vi "make_plot_projection.vi"(0 "Plot Scene Object In":refnum<vi>, 2 "Surface Mesh In":refnum<vi>, 3 "Minimum":T1, 7 "Data Mesh Object In":refnum<vi>, 8 "Projection Properties":T3, 9 "Contour Object In":refnum<vi>, 11 "Normals Object In":refnum<vi>, 13 "PL Object In":refnum<vi>) -> (14 "Plot Scene Object Out":refnum<vi>, 16 "Surface Mesh Out":refnum<vi>)   [LabVIEW 2020, in "3DPC_SurfacePlot.xctl"]
uses:
  <vilib>/Native 3D Graph/xcontrol/3DPC_SurfacePlot.xctl
  <vilib>/Native 3D Graph/typedefs/prop_plot_projection.ctl
  <vilib>/Native 3D Graph/typedefs/range_cluster.ctl
  <vilib>/Native 3D Graph/typedefs/min_max.ctl
  <vilib>/picture/3D Picture Control/Object/Create Object (name).vi
  <vilib>/picture/3D Picture Control/NI_3D Picture Control.lvlib
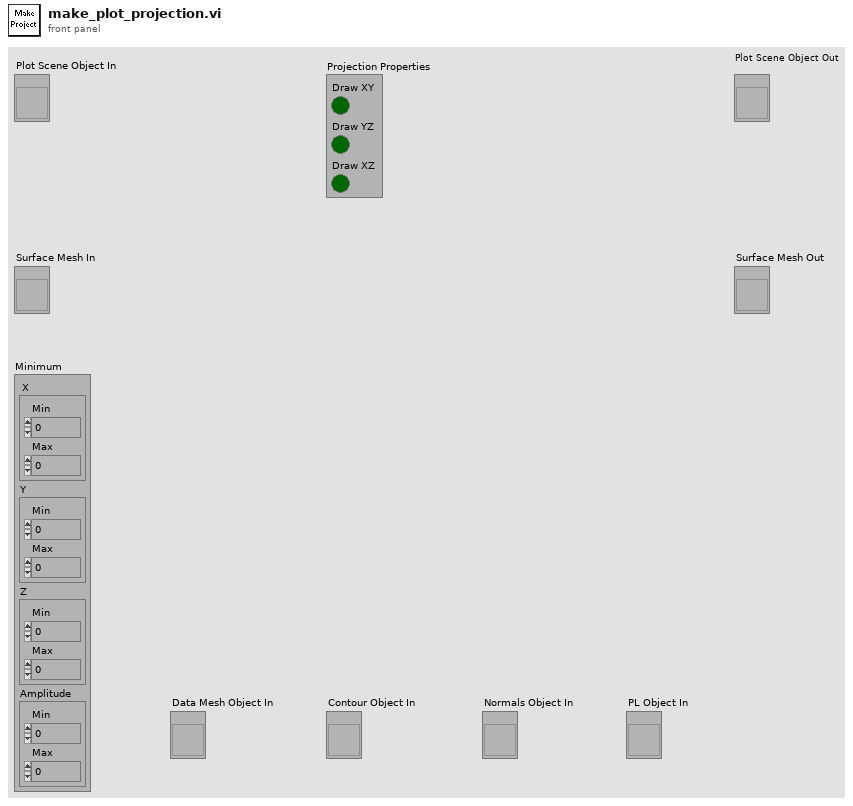
[diagram p1: front panel]
types:
  T1 = typedef "3DPC_SurfacePlot.xctl/range_cluster.ctl" = cluster{"X":T2, "Y":T2, "Z":T2, "Amplitude":T2}
  T2 = typedef "3DPC_SurfacePlot.xctl/min_max.ctl" = cluster{"Min":sgl, "Max":sgl}
  T3 = typedef "3DPC_SurfacePlot.xctl/prop_plot_projection.ctl" = cluster{"Draw XY":bool, "Draw YZ":bool, "Draw XZ":bool}
  T4 = enum16{"Inherit Value", "Points", "Wireframe", "Polygons"}
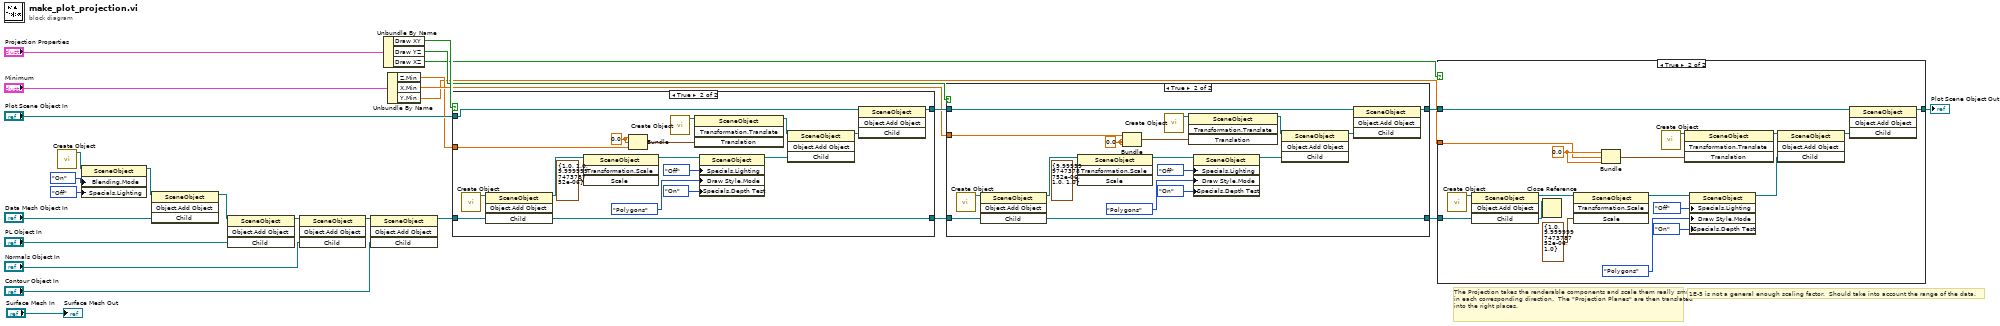
[diagram p0: block diagram]
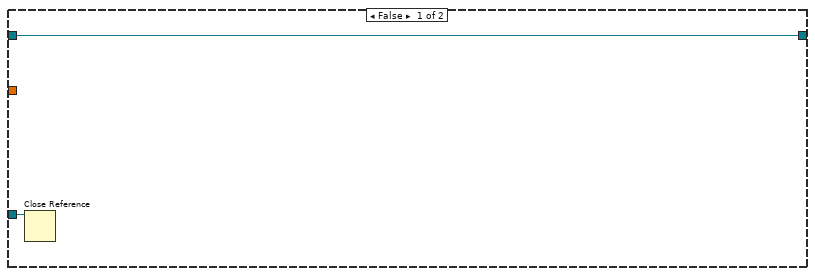
[diagram p2: hidden frame]
diagram:
  # "1E-5 is not a general enough scaling factor.  Should take into account the range of the data."
  # "The Projection takes the renderable components and scale them really small in each corresponding direction.  The \"Projection Planes\" are then translated into the right places."
  n1 = call-poly <vilib>:"Create Object.vi"() -> ("Scene:New Object"=w8:refnum<vi>)  [unwired: 10 in, 1 out]
  n2 = property class="SceneObject"(reference=w8, "Blending.Mode"=enum16{"Inherit Value", "Off", "On"}."On" ("Blending:Mode"), "Specials.Lighting"=enum16{"Inherit Value", "Off", "On"}."Off" ("Specials:Lighting")) -> (reference out=w9:refnum<vi>)  [unwired: 1 in, 1 out]
  n3 = invoke class="SceneObject" method="Object.Add Object"(reference=w9, "Child"="Data Mesh Object In") -> (reference out=w17:refnum<vi>)  [unwired: 2 in, 3 out]
  n4 = invoke class="SceneObject" method="Object.Add Object"(reference=w17, "Child"="PL Object In") -> (reference out=w16:refnum<vi>)  [unwired: 2 in, 3 out]
  n5 = invoke class="SceneObject" method="Object.Add Object"(reference=w16, "Child"="Normals Object In") -> (reference out=w15:refnum<vi>)  [unwired: 2 in, 3 out]
  n6 = invoke class="SceneObject" method="Object.Add Object"(reference=w15, "Child"="Contour Object In") -> (reference out=w10:refnum<vi>)  [unwired: 2 in, 3 out]
  n7 = Unbundle By Name("Projection Properties") -> ("Draw XY"=w21:bool, "Draw YZ"=w19:bool, "Draw XZ"=w18:bool)
  n8 = Unbundle By Name("Minimum") -> ("Z.Min"=w2:sgl, "X.Min"=w3:sgl, "Y.Min"=w1:sgl)
  n9 = case shown="True" w21 {
    tunnel: "Plot Scene Object In" -> [w29 w45]
    tunnel: [w29 w46] -> w24
    tunnel: [w28 w31] -> w25
    tunnel: w10 -> [w28 w32]
    tunnel: w2 -> [_ w30]
    frame False {
    }
    frame True {
      w36 = sgl 0.0 ("Minimum")
      n10 = call-poly <vilib>:"Create Object.vi"() -> ("Scene:New Object"=w47:refnum<vi>)  [unwired: 10 in, 1 out]
      n11 = invoke class="SceneObject" method="Object.Add Object"(reference=w47, "Child"=w32) -> (reference out=w41:refnum<vi>, "Child"=w31:refnum<vi>)  [unwired: 2 in, 2 out]
      n12 = invoke class="SceneObject" method="Transformation.Scale"(reference=w41, "Scale"=cluster{"X":sgl, "Y":sgl, "Z":sgl} {"X"=1.0, "Y"=1.0, "Z"=1e-05}) -> (reference out=w40:refnum<vi>)  [unwired: 2 in, 3 out]
      n13 = Bundle("Minimum"=w36, "Minimum"=w36, "Min"=w30) -> (w35:cluster{"Minimum":sgl, "Minimum":sgl, "Min":sgl})  [unwired: 1 out]
      n14 = call-poly <vilib>:"Create Object.vi"() -> ("Scene:New Object"=w38:refnum<vi>)  [unwired: 10 in, 1 out]
      n15 = invoke class="SceneObject" method="Transformation.Translate"(reference=w38, "Translation"=w35) -> (reference out=w37:refnum<vi>)  [unwired: 2 in, 3 out]
      n16 = property class="SceneObject"(reference=w40, "Specials.Lighting"=enum16{"Inherit Value", "Off", "On"}."Off" ("Specials:Lighting"), "Draw Style.Mode"=T4."Polygons" ("Draw Style:Mode"), "Specials.Depth Test"=enum16{"Inherit Value", "Off", "On"}."On" ("Specials:Depth Test")) -> (reference out=w34:refnum<vi>)  [unwired: 1 in, 1 out]
      n17 = invoke class="SceneObject" method="Object.Add Object"(reference=w37, "Child"=w34) -> (reference out=w33:refnum<vi>)  [unwired: 2 in, 3 out]
      n18 = invoke class="SceneObject" method="Object.Add Object"(reference=w45, "Child"=w33) -> (reference out=w46:refnum<vi>)  [unwired: 2 in, 3 out]
    }
  }
  n19 = case shown="True" w19 {
    tunnel: w24 -> [w49 w65]
    tunnel: [w49 w66] -> w22
    tunnel: w25 -> [w48 w61]
    tunnel: [w48 w55] -> w23
    tunnel: w3 -> [_ w50]
    frame False {
    }
    frame True {
      w51 = sgl 0.0 ("Minimum")
      n20 = call-poly <vilib>:"Create Object.vi"() -> ("Scene:New Object"=w67:refnum<vi>)  [unwired: 10 in, 1 out]
      n21 = invoke class="SceneObject" method="Object.Add Object"(reference=w67, "Child"=w61) -> (reference out=w60:refnum<vi>, "Child"=w55:refnum<vi>)  [unwired: 2 in, 2 out]
      n22 = invoke class="SceneObject" method="Transformation.Scale"(reference=w60, "Scale"=cluster{"X":sgl, "Y":sgl, "Z":sgl} {"X"=1e-05, "Y"=1.0, "Z"=1.0}) -> (reference out=w59:refnum<vi>)  [unwired: 2 in, 3 out]
      n23 = Bundle("Min"=w50, "Minimum"=w51, "Minimum"=w51) -> (w54:cluster{"Min":sgl, "Minimum":sgl, "Minimum":sgl})  [unwired: 1 out]
      n24 = call-poly <vilib>:"Create Object.vi"() -> ("Scene:New Object"=w53:refnum<vi>)  [unwired: 10 in, 1 out]
      n25 = invoke class="SceneObject" method="Transformation.Translate"(reference=w53, "Translation"=w54) -> (reference out=w52:refnum<vi>)  [unwired: 2 in, 3 out]
      n26 = property class="SceneObject"(reference=w59, "Specials.Lighting"=enum16{"Inherit Value", "Off", "On"}."Off" ("Specials:Lighting"), "Draw Style.Mode"=T4."Polygons" ("Draw Style:Mode"), "Specials.Depth Test"=enum16{"Inherit Value", "Off", "On"}."On" ("Specials:Depth Test")) -> (reference out=w57:refnum<vi>)  [unwired: 1 in, 1 out]
      n27 = invoke class="SceneObject" method="Object.Add Object"(reference=w52, "Child"=w57) -> (reference out=w56:refnum<vi>)  [unwired: 2 in, 3 out]
      n28 = invoke class="SceneObject" method="Object.Add Object"(reference=w65, "Child"=w56) -> (reference out=w66:refnum<vi>)  [unwired: 2 in, 3 out]
    }
  }
  n29 = case shown="True" w18 {
    tunnel: w22 -> [w69 w85]
    tunnel: [w69 w86] -> w20
    tunnel: w23 -> [w68 w81]
    tunnel: w1 -> [_ w70]
    frame False {
      n30 = Close Reference(reference=w68) -> ()  [unwired: 1 in, 1 out]
    }
    frame True {
      w71 = sgl 0.0 ("Minimum")
      n31 = call-poly <vilib>:"Create Object.vi"() -> ("Scene:New Object"=w87:refnum<vi>)  [unwired: 10 in, 1 out]
      n32 = invoke class="SceneObject" method="Object.Add Object"(reference=w87, "Child"=w81) -> (reference out=w80:refnum<vi>, "Child"=w75:refnum<vi>)  [unwired: 2 in, 2 out]
      n33 = Close Reference(reference=w75) -> ()  [unwired: 1 in, 1 out]
      n34 = invoke class="SceneObject" method="Transformation.Scale"(reference=w80, "Scale"=cluster{"X":sgl, "Y":sgl, "Z":sgl} {"X"=1.0, "Y"=1e-05, "Z"=1.0}) -> (reference out=w79:refnum<vi>)  [unwired: 2 in, 3 out]
      n35 = Bundle("Minimum"=w71, "Min"=w70, "Minimum"=w71) -> (w73:cluster{"Minimum":sgl, "Min":sgl, "Minimum":sgl})  [unwired: 1 out]
      n36 = call-poly <vilib>:"Create Object.vi"() -> ("Scene:New Object"=w74:refnum<vi>)  [unwired: 10 in, 1 out]
      n37 = invoke class="SceneObject" method="Transformation.Translate"(reference=w74, "Translation"=w73) -> (reference out=w72:refnum<vi>)  [unwired: 2 in, 3 out]
      n38 = property class="SceneObject"(reference=w79, "Specials.Lighting"=enum16{"Inherit Value", "Off", "On"}."Off" ("Specials:Lighting"), "Draw Style.Mode"=T4."Polygons" ("Draw Style:Mode"), "Specials.Depth Test"=enum16{"Inherit Value", "Off", "On"}."On" ("Specials:Depth Test")) -> (reference out=w77:refnum<vi>)  [unwired: 1 in, 1 out]
      n39 = invoke class="SceneObject" method="Object.Add Object"(reference=w72, "Child"=w77) -> (reference out=w76:refnum<vi>)  [unwired: 2 in, 3 out]
      n40 = invoke class="SceneObject" method="Object.Add Object"(reference=w85, "Child"=w76) -> (reference out=w86:refnum<vi>)  [unwired: 2 in, 3 out]
    }
  }
  "Plot Scene Object Out" <- w20
  "Surface Mesh Out" <- "Surface Mesh In"
